vi "View Insert VI.vi"(9 "UpdateInsertableVI":T1[](array[typedef]), 10 "Name":string, 11 "TabControl in":refnum<vi>) -> ()   [LabVIEW 2020, in "MDI ViewManager.lvlib"]
uses:
  MDI ViewManager.lvlib
  Typedef/Update ViewList.ctl
  <vilib>/Utility/miscctls.llb/LVBoundsTypeDef.ctl
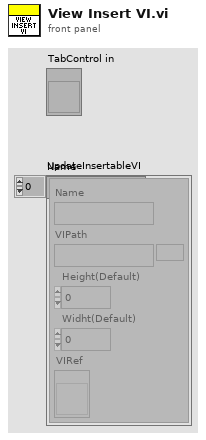
[diagram p1: front panel]
types:
  T1 = typedef "MDI ViewManager.lvlib/Update ViewList.ctl" = cluster{"Name":string, "VIPath":path, "Height(Default)":u32, "Widht(Default)":u32, "VIRef":refnum<vi>}
  T2 = typedef "LVBoundsTypeDef.ctl" = cluster{"Width":u32, "Height":u32}
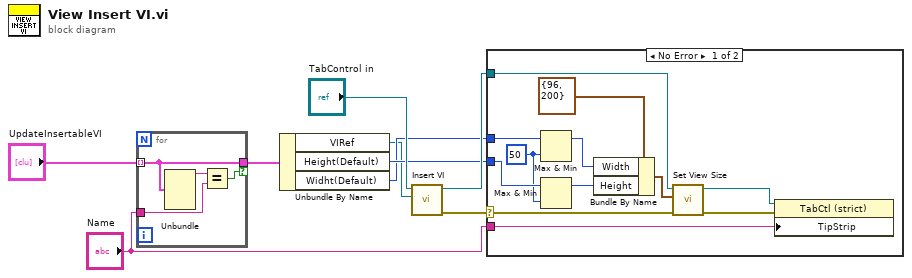
[diagram p0: block diagram]
diagram:
  n1 = for {
    tunnel: "UpdateInsertableVI" -> [w10] mode=indexing
    tunnel: "Name" -> [w13]
    tunnel: [w10] -> w4 if=w11
    n2 = Unbundle(w10) -> ("Name"=w12:string)  [unwired: 4 out]
    n3 = Equal?(x=w12, y=w13) -> (x = y?=w11:bool)
  }
  n4 = Unbundle By Name(w4) -> ("VIRef"=w1:refnum<vi>, "Height(Default)"=w3:u32, "Widht(Default)"=w2:u32)
  n5 = call "Insert VI.vi"("VIRef"=w1, "TabControl in"="TabControl in") -> ("error out"=w5:errorcluster, "TabControl out"=w6:refnum<vi>)  [unwired: 8 in]
  n6 = case shown="No Error" w5 {
    selector: w5 -> [w19 _]
    tunnel: "Name" -> [w22 _]
    tunnel: w6 -> [w21 _]
    tunnel: w3 -> [w25 _]
    tunnel: w2 -> [w24 _]
    frame No Error {
      w23 = u32 50 ("y")
      n7 = Max & Min(x=w24, y=w23) -> (max(x,y)=w15:u32)  [unwired: 1 out]
      n8 = Max & Min(x=w25, y=w23) -> (max(x,y)=w14:u32)  [unwired: 1 out]
      n9 = Bundle By Name(cluster=T2 {"Width"=96, "Height"=200} ("TabDimension"), "Width"=w15, "Height"=w14) -> (w16:T2)
      n10 = call "Set View Size.vi"("error in (no error)"=w19, "TabDimension"=w16, "TabControlRef in"=w21) -> ("error out"=w18:errorcluster, "TabControlRef out"=w20:refnum<vi>)  [unwired: 7 in]
      n11 = property class="TabCtl (strict)"(reference=w20, error in=w18, "TipStrip"=w22) -> ()  [unwired: 2 out]
    }
    frame Error {
    }
  }
